vi "find module index.vi"(8 "error in":errorcluster, 10 "module ID":string, 11 "Standard Engine Runtime in":refnum<class "Standard Engine Runtime.lvclass">) -> (0 "error out":errorcluster, 2 "index":i32, 3 "Standard Engine Runtime out":refnum<class "Standard Engine Runtime.lvclass">)   [LabVIEW 2013, in "Standard Engine Runtime.lvclass"]
uses:
  Standard Engine Runtime.lvclass
  Standard Engine Runtime.lvclass/Standard Engine Runtime.ctl
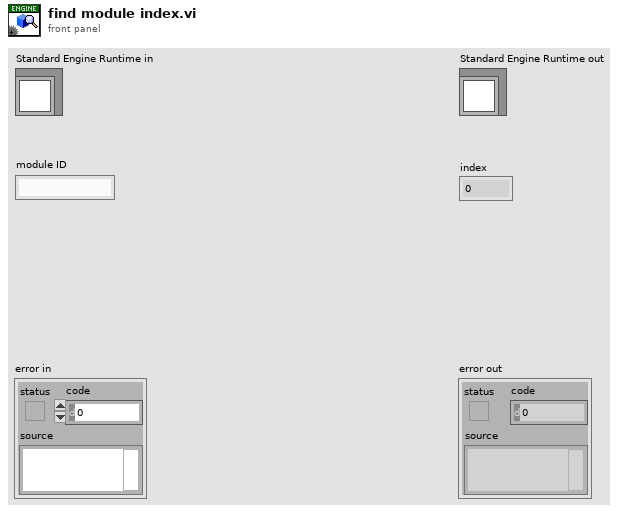
[diagram p1: front panel]
types:
  T1 = typedef "main engine.lvlib/shared engine config.ctl" = cluster{"main config":variant, "module IDs":string[]}
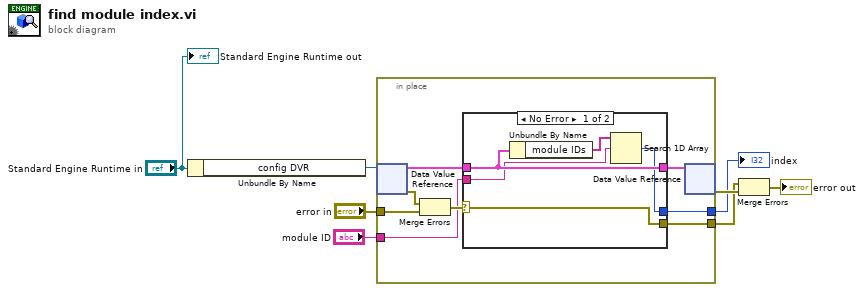
[diagram p0: block diagram]
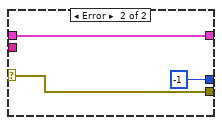
[diagram p2: hidden frame]
diagram:
  n1 = Unbundle By Name("Standard Engine Runtime in") -> ("config DVR"=w7:refnum<data-value>)
  n2 = in-place {
    in-place-border: "error in" -> [w16]
    in-place-border: [w11] -> w4
    in-place-border: [w10] -> w2
    in-place-border: "module ID" -> [w9]
    n3 = in-place-dvr #1(w7) -> (w12:T1, w15:errorcluster)
    n4 = Merge Errors(w15, w16) -> (w14:errorcluster)
    n5 = case shown="No Error" w14 {
      selector: w14 -> [w21 w24]
      tunnel: [w20 w23] -> w13
      tunnel: w12 -> [w20 w23]
      tunnel: [w21 w24] -> w11
      tunnel: [w17 -1] -> w10
      tunnel: w9 -> [w18 _]
      frame No Error {
        n6 = Unbundle By Name(w20) -> ("module IDs"=w19:string[])
        n7 = Search 1D Array(1D array=w19, element=w18) -> (index of element=w17:i32)  [unwired: 1 in]
      }
      frame Error {
      }
    }
    n8 = in-place-dvr #1(w13) -> (w5:errorcluster)  [unwired: 1 out]
  }
  "index" <- w2
  n9 = Merge Errors(w4, w5) -> (→"error out":errorcluster)
  "Standard Engine Runtime out" <- "Standard Engine Runtime in"
